vi "EditMeasurement.vi"(8 "error in (no error)":errorcluster, 9 "instrument measure":sgl, 10 "measurement id":u16, 11 "ByteGSAPIBase in":refnum<class "ByteGSAPIBase.lvclass">) -> (0 "error out":errorcluster, 2 "Measurement data":T1, 3 "ByteGSAPIBase out":refnum<class "ByteGSAPIBase.lvclass">)   [LabVIEW 2019, in "ByteGSWebAPI.lvlib" / "ByteGSAPIBase.lvclass"]
uses:
  ByteGSAPIBase.lvclass
  MeasurementResData.ctl
  <vilib>/Bytelabs/ByteREST/ByteRESTClass/ByteRESTBase/HTTP/Status_Code.ctl
  TypeDef/EditMeasurementReqData.ctl
  ByteGSAPIBase.lvclass/ByteGSAPIBase.ctl
  <vilib>/Bytelabs/ByteREST/ByteRESTClass/ByteRESTBase/RESTBase.lvclass
  <vilib>/numeric/Random Number (Range) U64.vi
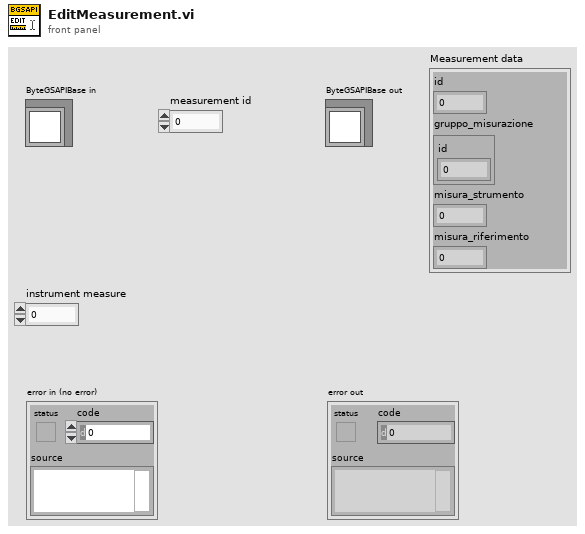
[diagram p1: front panel]
types:
  T1 = typedef "ByteGSWebAPI.lvlib/ByteGSAPIBase.lvclass/MeasurementResData.ctl" = cluster{"id":i32, "gruppo_misurazione":cluster{"id":i32}, "misura_strumento":dbl, "misura_riferimento":dbl}
  T2 = typedef "ByteGSWebAPI.lvlib/ByteGSAPIBase.lvclass/EditMeasurementReqData.ctl" = cluster{"Id_Group":i32, "misura_strumento":sgl, "misura_riferimento":sgl}
  T3 = typedef "ByteREST.lvlib/RESTBase.lvclass/Status_Code.ctl" = u16
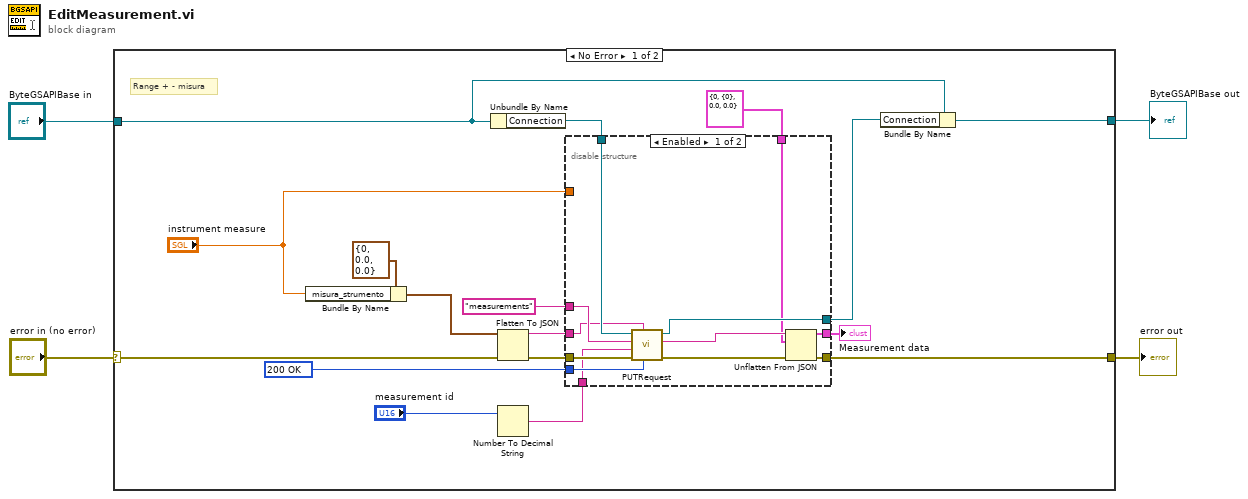
[diagram p0: block diagram]
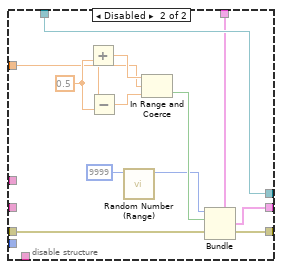
[diagram p2: hidden frame]
diagram:
  n1 = case shown="No Error" "error in (no error)" {
    selector: "error in (no error)" -> [w14 w47]
    tunnel: [w9 w47] -> w3
    tunnel: [w19 w46] -> w1
    tunnel: "ByteGSAPIBase in" -> [w21 w46]
    frame No Error {
      w16 = T3 200 items=["200 OK"=200, "201 Created"=201, "400 Bad Request"=400, "401 Unauthorized"=401, "403 Forbidden"=403, "404 Not Found"=404, "405 Method Not Allowed"=405, "406 Not Acceptable"=406, "500 Internal Server Error"=500] ("expected response")
      # "Range + - misura"
      n2 = Bundle By Name(cluster=T2 {"Id_Group"=0, "misura_strumento"=0.0, "misura_riferimento"=0.0} ("Valori"), "misura_strumento"="instrument measure") -> (w12:T2)
      n3 = Unbundle By Name(w21) -> ("Connection"=w20:refnum<class "RESTBase.lvclass">)
      n4 = Flatten To JSON(anything=w12, error in (no error)=w14) -> (JSON string=w11:string, 11:w13:errorcluster)  [unwired: 1 in]
      n5 = Number To Decimal String(number="measurement id") -> (decimal integer string=w6:string)  [unwired: 1 in]
      n6 = disable-structure shown="Enabled" {
        disable-tunnel: w20 -> [w33 w38]
        disable-tunnel: [w32 w38] -> w18
        disable-tunnel: "measurements" ("Request") -> [w31 _]
        disable-tunnel: w16 -> [w30 _]
        disable-tunnel: w13 -> [w29 w34]
        disable-tunnel: w11 -> [w28 _]
        disable-tunnel: T1 {"id"=0, "gruppo_misurazione"={"id"=0}, "misura_strumento"=0.0, "misura_riferimento"=0.0} -> [w25 w36]
        disable-tunnel: [w24 w40] -> w5
        disable-tunnel: [w23 w34] -> w9
        disable-tunnel: "instrument measure" -> [_ w42]
        disable-tunnel: w6 -> [w22 _]
        frame Enabled {
          n7 = call-dynamic "PUTRequest.vi"("expected response"=w30, "Body in"=w28, "error in (no error)"=w29, "Parameter"=w22, "Request"=w31, "ByteRESTBase in"=w33) -> ("error out"=w26:errorcluster, "Body"=w27:string, "ByteRESTBase out"=w32:refnum<class "RESTBase.lvclass">)  [unwired: 2 in, 1 out]
          n8 = Unflatten From JSON(JSON string=w27, type and defaults=w25, error in (no error)=w26) -> (value=w24:T1, error out=w23:errorcluster)  [unwired: 4 in]
        }
        frame Disabled {
          w43 = 0.5
          n9 = Subtract(y=w43) -> (x=w41:dbl, x-y=w45:dbl)
          n10 = Add(x=w41, y=w43) -> (x+y=w44:dbl)
          n11 = call-poly <vilib>:"Random Number (Range).vi"("upper bound (100)"=u64 9999) -> ("number"=w35:u64)  [unwired: 10 in]
          n12 = In Range and Coerce(upper limit=w44, x=w42, lower limit=w45) -> (In Range?=w39:bool)  [unwired: 1 out]
          n13 = Bundle(cluster=w36, "id"=w35, "gruppo_misurazione"=w39) -> (w40:T1)  [unwired: 2 in]
        }
      }
      "Measurement data" <- w5
      n14 = Bundle By Name(cluster=w21, "Connection"=w18) -> (w19:refnum<class "ByteGSAPIBase.lvclass">)
    }
    frame Error {
    }
  }
  "error out" <- w3
  "ByteGSAPIBase out" <- w1
